vi "Write Scaled Data.vi"(8 "error in (no error)":errorcluster, 9 "Scaled Data":dbl[](array[numeric]), 10 "Parameters":string[](array[string]), 11 "1553 Component in":refnum<class "1553 Component.lvclass">) -> (0 "error out":errorcluster, 3 "1553 Component out":refnum<class "1553 Component.lvclass">)   [LabVIEW 2020, in "BCI-1553 API.lvlib" / "1553 Component.lvclass"]
doc: "Writes new scaled data to a set of configured parameters for this component. The data will be pushed to hardware memory depending on the configured scaling information."
uses:
  1553 Component.lvclass
  1553 Component.lvclass/1553 Component.ctl
  1553 SubComponent/1553 SubComponent.lvclass
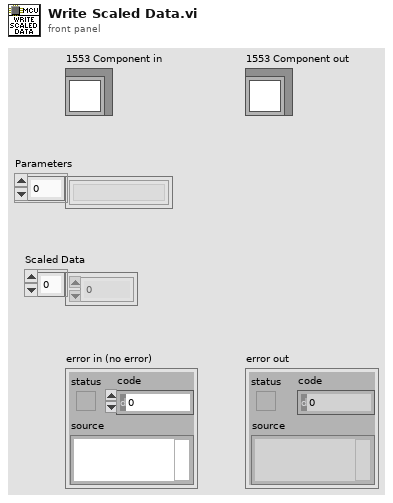
[diagram p1: front panel]
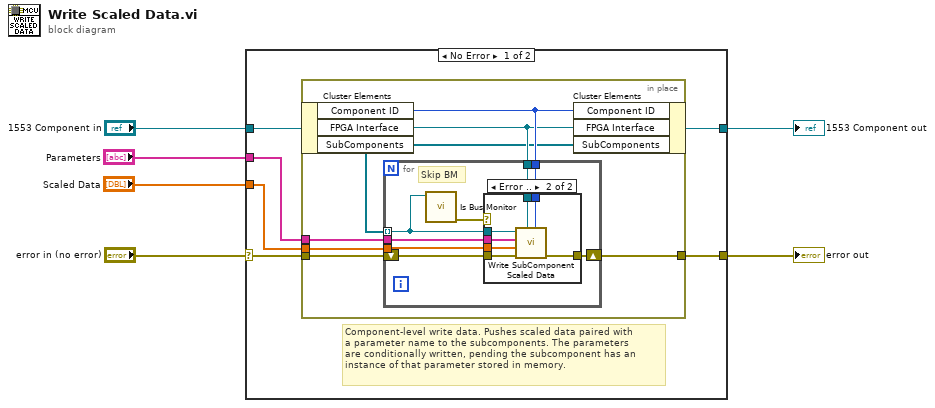
[diagram p0: block diagram]
diagram:
  n1 = case shown="No Error" "error in (no error)" {
    selector: "error in (no error)" -> [w11 w36]
    tunnel: [w10 w37] -> w4
    tunnel: "1553 Component in" -> [w12 w37]
    tunnel: "Parameters" -> [w9 _]
    tunnel: "Scaled Data" -> [w8 _]
    tunnel: [w7 w36] -> w1
    frame No Error {
      # "Component-level write data. Pushes scaled data paired with\na parameter name to the subcomponents. The parameters\nare conditionally written, pending the subcomponent has an\ninstance of that parameter stored in memory."
      n2 = in-place {
        in-place-border: w11 -> [w17]
        in-place-border: w9 -> [w16]
        in-place-border: w8 -> [w15]
        in-place-border: [w13] -> w7
        n3 = in-place-cluster #1(w12) -> ("Component ID"=w19:u8, "FPGA Interface"=w18:refnum<class "FPGA Interface.lvclass">, "SubComponents"=w14:refnum<class "1553 SubComponent.lvclass">[])
        n4 = for {
          tunnel: w14 -> [w21] mode=indexing
          tunnel: w19 -> [w26]
          tunnel: w18 -> [w27]
          tunnel: w16 -> [w24]
          tunnel: w15 -> [w23]
          shift-right: [w22] -> w13
          shift-left: w17 -> [w25]
          # "Skip BM"
          n5 = call "Is Bus Monitor.vi"("1553 SubComponent"=w21) -> ("error out"=w20:errorcluster)  [unwired: 10 in]
          n6 = case shown="Error .." w20 {
            tunnel: w21 -> [_ w35]
            tunnel: w27 -> [_ w34]
            tunnel: w26 -> [_ w33]
            tunnel: w25 -> [w28 w32]
            tunnel: w24 -> [_ w31]
            tunnel: w23 -> [_ w30]
            tunnel: [w28 w29] -> w22
            frame No Error {
            }
            frame Error {
              n7 = call-dynamic "Write SubComponent Scaled Data.vi"("Component ID"=w33, "FPGA Interface"=w34, "error in (no error)"=w32, "Scaled Data"=w30, "Parameters"=w31, "1553 SubComponent in"=w35) -> ("error out"=w29:errorcluster)  [unwired: 5 in]
            }
          }
        }
        n8 = in-place-cluster #1("Component ID"=w19, "FPGA Interface"=w18, "SubComponents"=w14) -> (w10:refnum<class "1553 Component.lvclass">)
      }
    }
    frame Error {
    }
  }
  "error out" <- w1
  "1553 Component out" <- w4
